vi "sort db drop data.vi"(8 "error in":errorcluster caption="error out", 10 "recordset data":variant[][](array[variant])=[variant, variant, variant, variant, variant, variant, variant, variant, variant, variant, variant, variant, variant, variant, variant, variant, variant, variant], 11 "add holder":T1) -> (0 "error out":errorcluster, 3 "cathode data":string[](array[string]))   [LabVIEW 2016]
doc: "Finds values in rose database and allows holder data to be dragged into the run order"
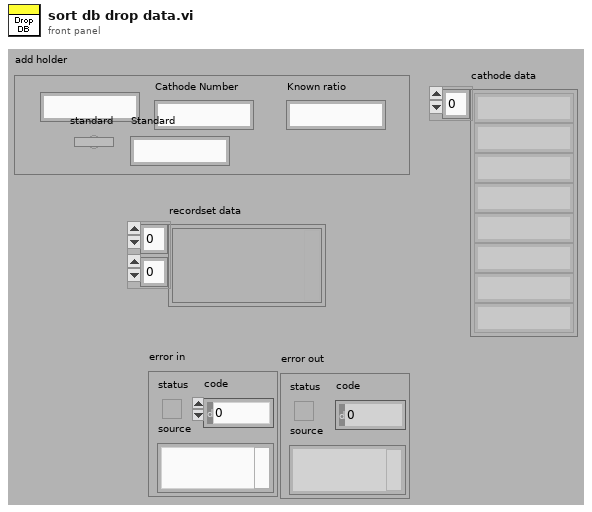
[diagram p1: front panel]
types:
  T1 = cluster{"position":string, "Cathode Number":string, "standard":bool, "Known ratio":string, "Standard":string}
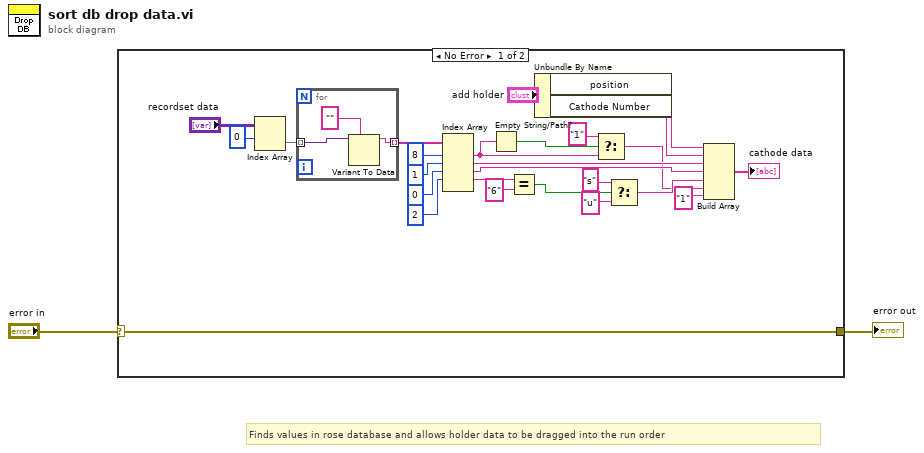
[diagram p0: block diagram]
diagram:
  # "Finds values in rose database and allows holder data to be dragged into the run order"
  n1 = case shown="No Error" "error in" {
    selector: "error in" -> [w3 w32]
    tunnel: [w3 w32] -> w1
    frame No Error {
      n2 = Index Array(array="recordset data", index (row)=0 ("disabled index (col)")) -> (element=w27:variant[])  [unwired: 1 in]
      n3 = for {
        tunnel: w27 -> [w31] mode=indexing
        tunnel: [w29] -> w22 mode=indexing
        n4 = Variant To Data(type="", Variant=w31) -> (data=w29:string)  [unwired: 1 in, 1 out]
      }
      n5 = Index Array(array=w22, index #1=8 ("index"), index #2=1 ("index"), index #3=0 ("index"), index #4=2 ("index")) -> (element #1=w24:string, element #2=w14:string, element #3=w13:string, element #4=w12:string)  [unwired: 1 in, 1 out]
      n6 = Empty String/Path?(string/path=w24) -> (empty?=w25:bool)
      n7 = Equal?(x=w12, y="6") -> (x = y?=w10:bool)
      n8 = Unbundle By Name("add holder") -> ("position"=w16:string, "Cathode Number"=w15:string)
      n9 = Select(t="1", s=w25, f=w24) -> (s? t:f=w6:string)
      n10 = Select(t="s", s=w10, f="u" ("t")) -> (s? t:f=w8:string)
      n11 = Build Array(w16, w15, w14, w13, w8, w6, "1" ("element")) -> (→"cathode data":string[])
    }
    frame Error {
    }
  }
  "error out" <- w1
